vi "Find NI-SWITCH Custom Device by Name.vi"(8 "error in":errorcluster, 10 "name":string, 11 "target in":refnum<k24>) -> (0 "error out":errorcluster, 2 "ni-switch custom device":T1=18446744073709551615 format="%.0x", 3 "target out":refnum<k24>)   [LabVIEW 2019, in "NI-SWITCH Scripting.lvlib"]
doc: "Returns the NI-SWITCH custom device with the specified name."
uses:
  NI-SWITCH Scripting.lvlib
  NationalInstruments.VeriStand.SystemDefinitionAPI
  <vilib>/NI VeriStand/Custom Device API/Custom Device Item Ref.ctl
  Shared/Constants.vi
  Shared/NI-SWITCH Shared.lvlib
  <vilib>/NI VeriStand/Custom Device API/Custom Device API.lvlib
panel:
  in  "error message":string="The item with the specified name is not an NI-SWITCH custom device."
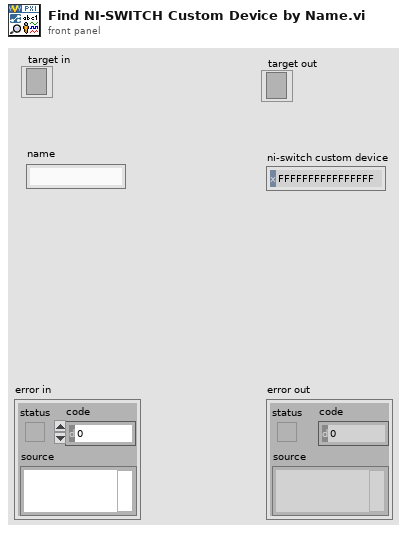
[diagram p1: front panel]
types:
  T1 = typedef "Custom Device API.lvlib/Custom Device Item Ref.ctl" = u64
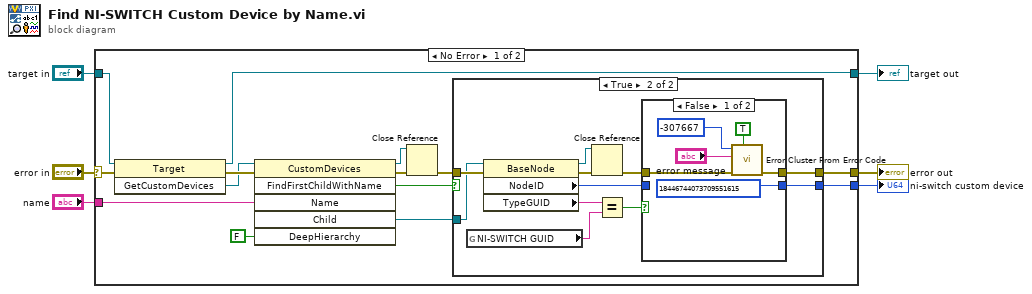
[diagram p0: block diagram]
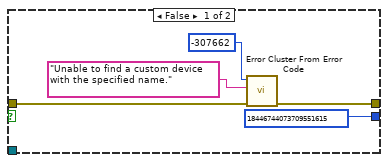
[diagram p2: hidden frame]
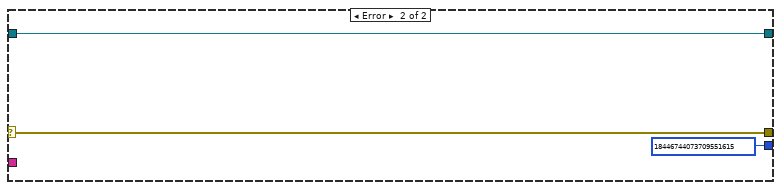
[diagram p4: hidden frame]
diagram:
  n1 = case shown="No Error" "error in" {
    selector: "error in" -> [w20 w47]
    tunnel: [w12 w47] -> w6
    tunnel: "target in" -> [w19 w46]
    tunnel: [w13 w46] -> w3
    tunnel: "name" -> [w10 _]
    tunnel: [w7 T1 18446744073709551615 ("ni-switch custom device")] -> w1
    frame No Error {
      n2 = invoke class="Target" method="GetCustomDevices"(reference=w19, error in=w20) -> (reference out=w13:refnum<k24>, error out=w18:errorcluster, "GetCustomDevices"=w17:refnum<k24>)  [unwired: 1 in]
      n3 = invoke class="CustomDevices" method="FindFirstChildWithName"(reference=w17, error in=w18, "Name"=w10, "DeepHierarchy"=FALSE) -> (reference out=w16:refnum<k24>, error out=w15:errorcluster, "FindFirstChildWithName"=w8:bool, "Child"=w9:refnum<k24>)  [unwired: 2 in, 2 out]
      n4 = Close Reference(reference=w16, error in (no error)=w15) -> (error out=w14:errorcluster)
      n5 = case shown="True" w8 {
        tunnel: w14 -> [w24 w36]
        tunnel: [w23 w26] -> w12
        tunnel: w9 -> [_ w34]
        tunnel: [T1 18446744073709551615 ("ni-switch custom device") w28] -> w7
        frame False {
          n6 = call <vilib>:"Error Cluster From Error Code.vi"("error in (no error)"=w24, "error message (\"\")"="Unable to find a custom device with the specified name." ("error message (\"\")"), "error code (0)"=-307662) -> ("error out"=w23:errorcluster)  [unwired: 6 in]
        }
        frame True {
          n7 = global read "Constants.vi" "NI-SWITCH GUID"() -> (w30:string)
          n8 = property class="BaseNode"(reference=w34, error in=w36) -> (reference out=w33:refnum<k24>, error out=w35:errorcluster, "NodeID"=w29:u64, "TypeGUID"=w31:string)
          n9 = Close Reference(reference=w33, error in (no error)=w35) -> (error out=w27:errorcluster)
          n10 = Equal?(x=w31, y=w30) -> (x = y?=w32:bool)
          n11 = case shown="False" w32 {
            tunnel: w29 -> [_ w44]
            tunnel: [T1 18446744073709551615 ("ni-switch custom device") w44] -> w28
            tunnel: w27 -> [w40 w43]
            tunnel: [w39 w43] -> w26
            frame False {
              n12 = call <vilib>:"Error Cluster From Error Code.vi"("show call chain? (False)"=TRUE, "error in (no error)"=w40, "error message (\"\")"="error message", "error code (0)"=-307667) -> ("error out"=w39:errorcluster)  [unwired: 5 in]
            }
            frame True {
            }
          }
        }
      }
    }
    frame Error {
    }
  }
  "target out" <- w3
  "error out" <- w6
  "ni-switch custom device" <- w1
